vi "waveformgraph2.vi"() -> ()   [LabVIEW 2015]
uses:
  <vilib>/Analysis/baseanly.llb/Mean (DBL).vi
  <vilib>/Analysis/NI_AALBase.lvlib
panel:
  in  "Path":path
  out "Multiwaveform Graph":dbl[][](graph)
  out "Waveform Chart":dbl(graph)
  in  "stop":bool
  out "Ultimos datos":cluster{i32, dbl, dbl[]}(graph)
  out "Todos los datos":dbl[](graph)
  in  "Total de muestras":i32
  out "Valor minimo":dbl
  out "Valor maximo":dbl
  out "Promedio":dbl
  in  "Numero de las ultimas \nmuestras representadas":i32
  out "String":string
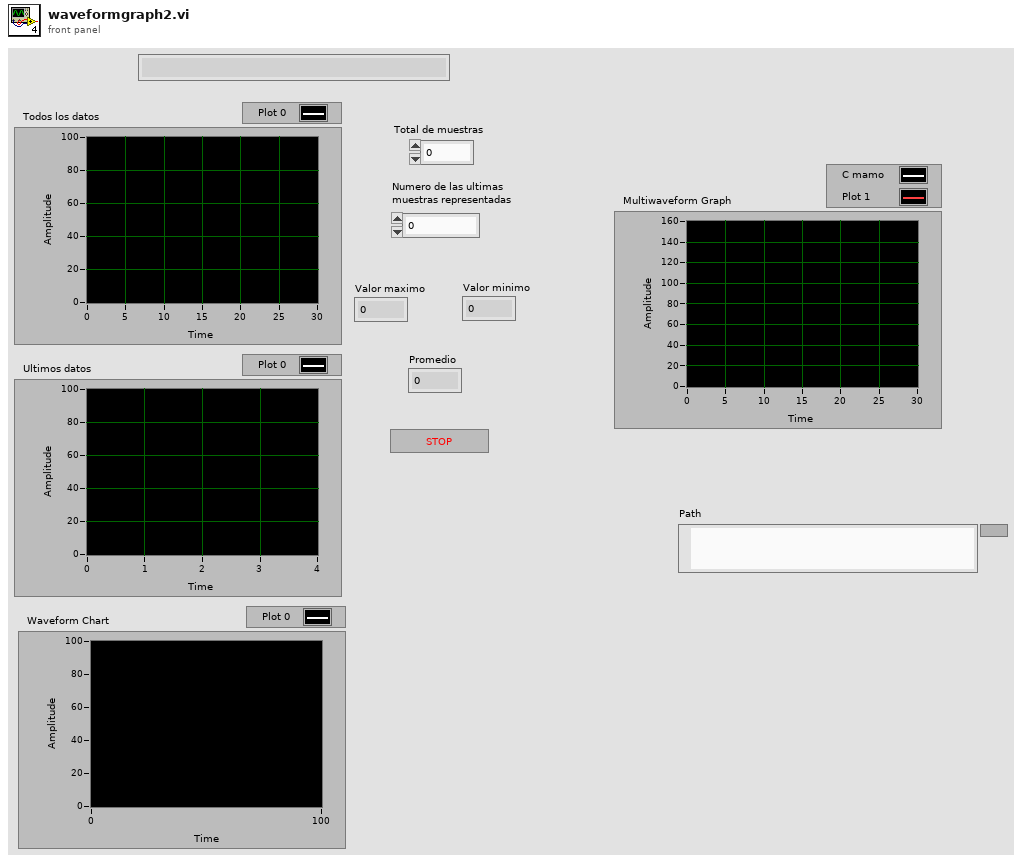
[diagram p1: front panel]
types:
  T1 = typedef "NI_Matrix.lvlib/RealMatrix.ctl" = dbl[][]
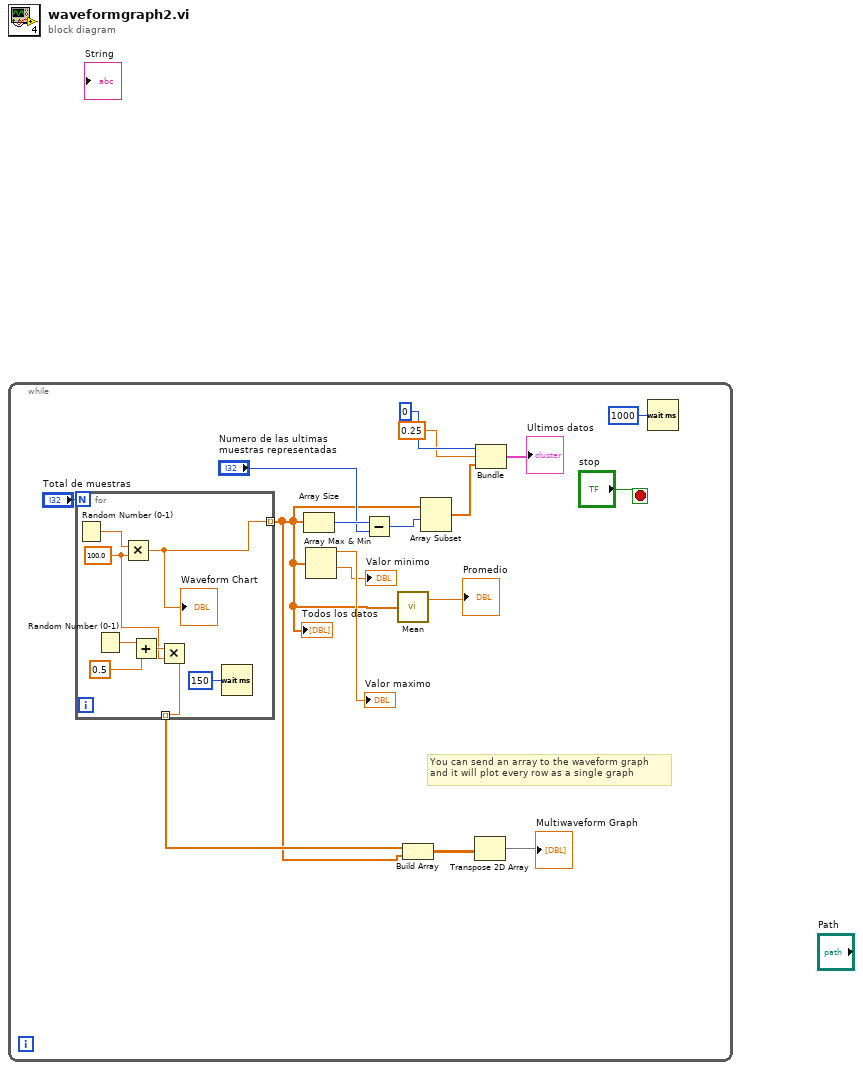
[diagram p0: block diagram]
diagram:
  n1 = while {
    stop <- "stop" stop-if-true
    # "You can send an array to the waveform graph\nand it will plot every row as a single graph"
    n2 = for {
      N: "Total de muestras" -> [_]
      tunnel: [w24] -> w3 mode=indexing
      tunnel: [w18] -> w4 mode=indexing
      w19 = 100.0 ("y")
      n3 = Random Number (0-1)() -> (number: 0 to 1=w25:dbl)
      n4 = Random Number (0-1)() -> (number: 0 to 1=w22:dbl)
      n5 = Multiply(x=w25, y=w19) -> (x*y=w24:dbl)
      "Waveform Chart" <- w24
      n6 = Add(x=w22, y=0.5) -> (x+y=w20:dbl)
      n7 = Multiply(x=w20, y=w19) -> (x*y=w18:dbl)
      n8 = Wait (ms)(milliseconds to wait=u32 150) -> ()  [unwired: 1 out]
    }
    "Todos los datos" <- w3
    n9 = Array Size(array=w3) -> (size(s)=w15:i32)
    n10 = Array Max & Min(array=w3) -> (max value=→"Valor maximo":dbl, min value=→"Valor minimo":dbl)  [unwired: 2 out]
    n11 = Subtract(x=w15, y="Numero de las ultimas \nmuestras representadas") -> (x-y=w13:i32)
    n12 = call-poly <vilib>:"Mean.vi"("X"=w3) -> ("mean"=→"Promedio":dbl)  [unwired: 1 out]
    n13 = Build Array(w4, w3) -> (w2:T1)
    n14 = Array Subset(array=w3, index=w13) -> (w5:dbl[])  [unwired: 1 in]
    n15 = Transpose 2D Array(2D array=w2) -> (transposed array=→"Multiwaveform Graph":T1)
    n16 = Bundle(0, 0.25, w5) -> (→"Ultimos datos":cluster{i32, dbl, dbl[]})  [unwired: 1 in]
    n17 = Wait (ms)(milliseconds to wait=u32 1000) -> ()  [unwired: 1 out]
  }
